vi "CMI ADS127L21 - Merge Errors.vi"(1 "errors in":errorcluster[](array[cluster]), 2 "error in (no error)":errorcluster) -> (0 "error out":errorcluster)   [LabVIEW 2020]
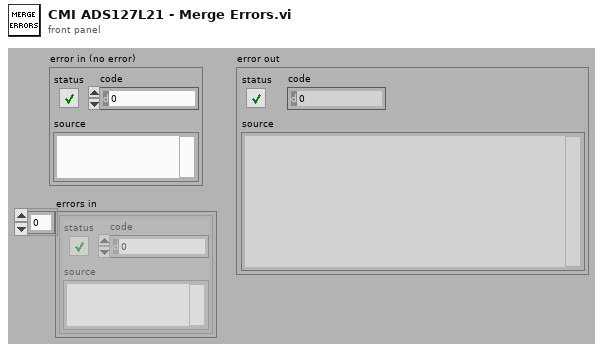
[diagram p1: front panel]
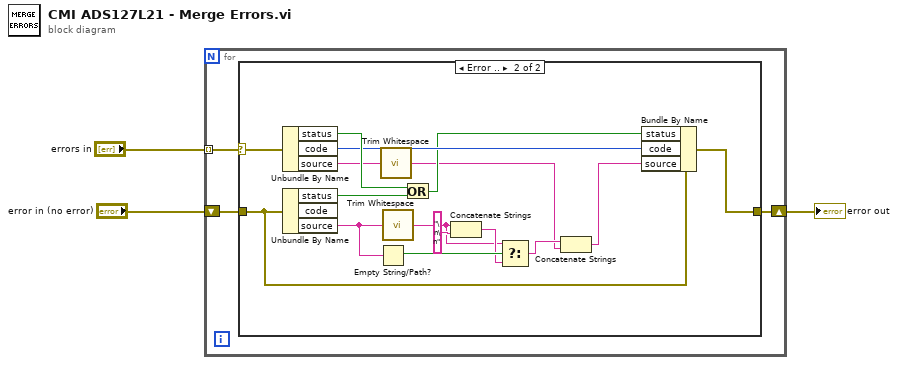
[diagram p0: block diagram]
diagram:
  n1 = for {
    tunnel: "errors in" -> [w6] mode=indexing
    shift-right: [w4] -> w1
    shift-left: "error in (no error)" -> [w5]
    n2 = case shown="Error .." w6 {
      selector: w6 -> [_ w23]
      tunnel: w5 -> [w7 w20]
      tunnel: [w7 w8] -> w4
      frame No Error {
      }
      frame Error {
        n3 = Unbundle By Name(w23) -> ("status"=w22:bool, "code"=w19:i32, "source"=w11:string)
        n4 = Unbundle By Name(w20) -> ("status"=w21:bool, "source"=w16:string)  [unwired: 1 out]
        n5 = Empty String/Path?(string/path=w16) -> (empty?=w17:bool)
        n6 = call <vilib>:"Trim Whitespace.vi"("string"=w11) -> ("trimmed string"=w10:string)  [unwired: 1 in]
        n7 = call <vilib>:"Trim Whitespace.vi"("string"=w16) -> ("trimmed string"=w13:string)  [unwired: 1 in]
        n8 = Or(x=w22, y=w21) -> (x .or. y?=w18:bool)
        n9 = Concatenate Strings(w13, "\n\n" ("string")) -> (w15:string)
        n10 = Select(t=w13, s=w17, f=w15) -> (s? t:f=w12:string)
        n11 = Concatenate Strings(w12, w10) -> (w9:string)
        n12 = Bundle By Name(cluster=w20, "status"=w18, "code"=w19, "source"=w9) -> (w8:errorcluster)
      }
    }
  }
  "error out" <- w1
